vi "SegmentedLineEdge_Create.vi"(0 "reference":refnum<class "SegmentedLineEdge.lvclass">, 5 "error in (no error)":errorcluster) -> (14 "reference out":refnum<class "SegmentedLineEdge.lvclass">, 19 "error out":errorcluster)   [LabVIEW 2020, in "SegmentedLineEdge.lvclass"]
doc: "Creates and initializes a new SegmentedLineEdge object.\n\nThis object should be destroyed using a SegmentedLineEdge destructor VI or a virtual base class destructor VI.\n\n[GOOP 2.1]"
uses:
  <resource>/Framework/Providers/Open_GDS/UML/SegmentedLineEdge_class/SegmentedLineEdge.lvclass
  C:/Program Files (x86)/National Instruments/LabVIEW 2020/resource/Framework/Providers/Open_GDS/UML/GeneralPathEdge_class/GeneralPathEdge.lvclass
  <resource>/Framework/Providers/Open_GDS/UML/ArrowHead_class/ArrowHeadType.ctl
  <resource>/Framework/Providers/Open_GDS/UML/LineStyle_class/LineStyleType.ctl
  <resource>/Framework/Providers/Open_GDS/UML/GeneralPathEdge_class/GeneralPathEdge.lvclass
  <resource>/Framework/Providers/Open_GDS/UML/LineStyle_class/LineStyle.lvclass
  <resource>/Framework/Providers/Open_GDS/UML/ArrowHead_class/ArrowHead.lvclass
panel:
  # "The input reference should only\nbe wired when this method is called\nby a sub class constructor."
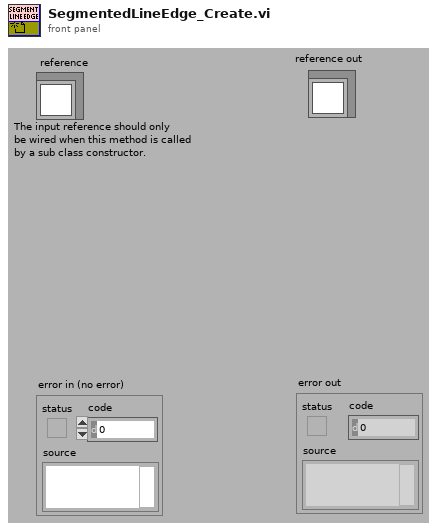
[diagram p1: front panel]
types:
  T1 = typedef "LineStyle.lvclass/LineStyleType.ctl" = enum16{"SOLID", "DOTTED"}
  T2 = typedef "ArrowHead.lvclass/ArrowHeadType.ctl" = enum16{"NONE", "TRIANGLE", "BLACK_TRIANGLE", "V", "HALF_V", "DIAMOND", "BLACK_DIAMOND"}
  T3 = typedef "SegmentedLineEdge.lvclass/ObjectAttributes.ctl" = cluster{"lineStyle":refnum<class "LineStyle.lvclass">, "startArrowHead":refnum<class "ArrowHead.lvclass">, "endArrowHead":refnum<class "ArrowHead.lvclass">, "startLabel":string, "midLabel":string, "endLabel":string, "MidLabelOffset":T4, "SplitWire":bool}
  T4 = typedef "Point Point2D.ctl" = cluster{"x":dbl, "y":dbl}
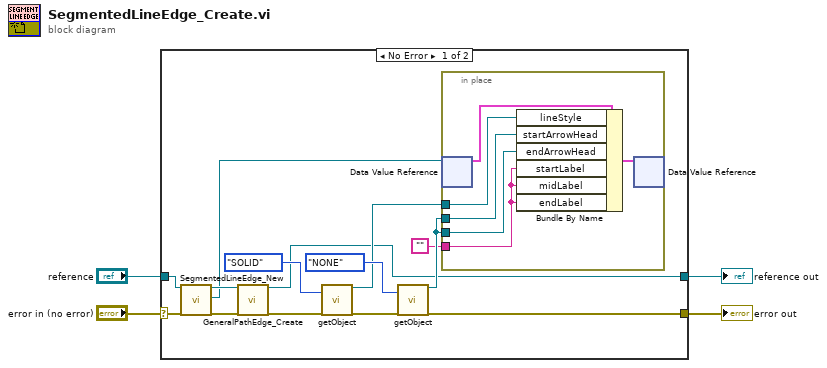
[diagram p0: block diagram]
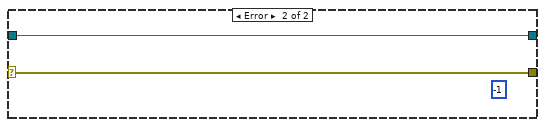
[diagram p2: hidden frame]
diagram:
  n1 = case shown="No Error" "error in (no error)" {
    selector: "error in (no error)" -> [w18 w26]
    tunnel: [w5 w25] -> w4
    tunnel: [w6 w26] -> w3
    tunnel: "reference" -> [w17 w25]
    frame No Error {
      n2 = call <resource>:"SegmentedLineEdge_New.vi"("reference in"=w17, "error in (no error)"=w18) -> ("reference out"=w15:refnum<class "SegmentedLineEdge.lvclass">, "DVRRefOut"=w7:refnum<data-value>, "error out"=w16:errorcluster)  [unwired: 2 in, 13 out]
      n3 = call <resource>:"GeneralPathEdge_Create.vi"("reference"=w15, "error in (no error)"=w16) -> ("reference out"=w5:refnum<class "SegmentedLineEdge.lvclass">, "error out"=w14:errorcluster)  [unwired: 1 in, 15 out]
      n4 = call <resource>:"getObject.vi"("lineStyle"=LineStyleType."SOLID", "error in (no error)"=w14) -> ("reference out"=w10:refnum<class "LineStyle.lvclass">, "error out"=w13:errorcluster)  [unwired: 16 out]
      n5 = call <resource>:"getObject.vi"("arrowHead"=ArrowHeadType."NONE", "error in (no error)"=w13) -> ("reference out"=w9:refnum<class "ArrowHead.lvclass">, "error out"=w6:errorcluster)  [unwired: 16 out]
      n6 = in-place {
        in-place-border: w10 -> [w23]
        in-place-border: w9 -> [w22]
        in-place-border: w9 -> [w21]
        in-place-border: "" -> [w20]
        n7 = in-place-dvr #1(w7) -> (w24:T3)  [unwired: 1 out]
        n8 = Bundle By Name(cluster=w24, "lineStyle"=w23, "startArrowHead"=w22, "endArrowHead"=w21, "startLabel"=w20, "midLabel"=w20, "endLabel"=w20) -> (w19:T3)
        n9 = in-place-dvr #1(w19) -> ()  [unwired: 2 out]
      }
    }
    frame Error {
      (unwired) -1 ("Nr of open handles")
    }
  }
  "error out" <- w3
  "reference out" <- w4
